vi "_ClassMethodsInheritance_Interface.vi"(9 "EventsIn":T1, 10 "Events":T2) -> ()   [LabVIEW 2013, in "ClassMethodsInheritance.lvclass"]
uses:
  ClassMethodsInheritance.lvclass
  <resource>/Framework/Providers/Veritech_LVCM/Support/Framework/_Plugins/_LVCMPlugin/_LVCMPlugin_EventsOut.ctl
  <resource>/Framework/Providers/Veritech_LVCM/Support/Framework/_Plugins/_LVCMPlugin/_LVCMPlugin_EventsIn.ctl
  <resource>/Framework/Providers/Veritech_LVCM/Support/Framework/_Plugins/_LVCMPlugin/_LVCMPlugin.lvclass
panel:
  in  "Multicolumn Listbox":i32(listbox)
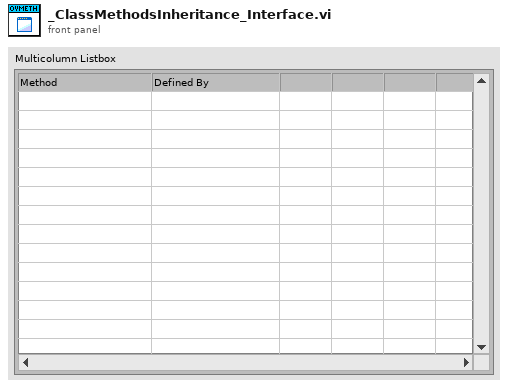
[diagram p1: front panel]
types:
  T1 = typedef "_LVCMPlugin.lvclass/_LVCMPlugin_EventsIn.ctl" = cluster{"Stop":refnum<user-event>, "Activate":refnum<user-event>}
  T2 = typedef "_LVCMPlugin.lvclass/_LVCMPlugin_EventsOut.ctl" = cluster{"ItemEdited":refnum<user-event>}
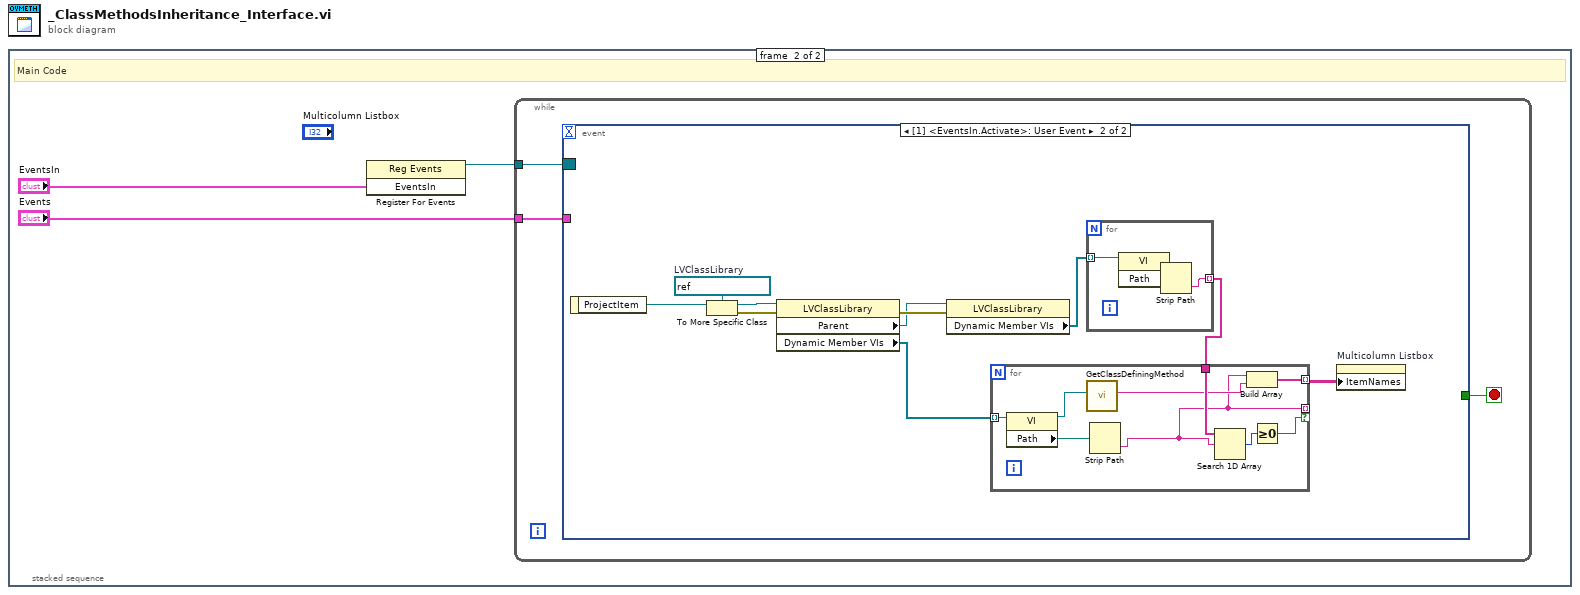
[diagram p0: block diagram]
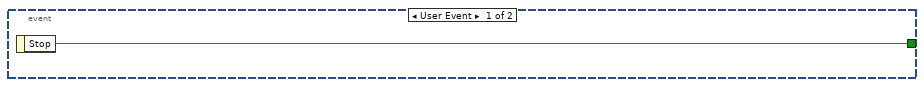
[diagram p3: hidden frame]
diagram:
  n1 = stacked-sequence {
    frame #0 {
      # "Init"
    }
    frame #1 {
      # "Main Code"
      n2 = register-events("EventsIn") -> (reference out=w2:refnum<event-registration>)  [unwired: 2 in, 1 out]
      n3 = while {
        tunnel: w2 -> [w6]
        tunnel: "Events" -> [w5]
        stop <- w4 stop-if-true
        n4 = event shown="[1] <EventsIn.Activate>: User Event" {
          selector: w6 -> [_ _]
          dyn-events: _ -> [_ _]
          timeout: _ -> [_ _]
          tunnel: w5 -> [_ _]
          tunnel: [w7 _] -> w4
          event User Event {
            n5 = event-data() -> ("Stop"=w7:bool)  [unwired: 1 in]
          }
          event User Event {
            w17 = refnum<vi> refnum  # LVClassLibrary
            n6 = event-data() -> ("ProjectItem"=w16:refnum<vi>)  [unwired: 1 in]
            n7 = To More Specific Class(target class=w17, reference=w16) -> (specific class reference=w15:refnum<vi>, error out=w14:errorcluster)  [unwired: 1 in]
            n8 = property class="LVClassLibrary"(reference=w15, error in=w14) -> (error out=w13:errorcluster, "Parent"=w8:refnum<vi>, "Dynamic Member VIs"=w12:refnum<vi>[])  [unwired: 1 out]
            n9 = property class="LVClassLibrary"(reference=w8, error in=w13) -> ("Dynamic Member VIs"=w11:refnum<vi>[])  [unwired: 2 out]
            n10 = for {
              tunnel: w11 -> [w20] mode=indexing
              tunnel: [w18] -> w10 mode=indexing
              n11 = property class="VI"(reference=w20) -> ("Path"=w19:path)  [unwired: 1 in, 2 out]
              n12 = Strip Path(path=w19) -> (name=w18:string)  [unwired: 1 out]
            }
            n13 = for {
              tunnel: w12 -> [w29] mode=indexing
              tunnel: w10 -> [w28]
              tunnel: [w22] -> _ mode=indexing if=w25
              tunnel: [w21] -> w9 mode=indexing
              n14 = property class="VI"(reference=w29) -> (reference out=w24:refnum<vi>, "Path"=w26:path)  [unwired: 1 in, 1 out]
              n15 = call "GetClassDefiningMethod.vi"("MethodVI"=w24) -> ("DefiningClass"=w23:string)  [unwired: 9 in, 1 out]
              n16 = Strip Path(path=w26) -> (name=w22:string)  [unwired: 1 out]
              n17 = Search 1D Array(1D array=w28, element=w22) -> (index of element=w27:i32)  [unwired: 1 in]
              n18 = Build Array(w22, w23) -> (w21:string[])
              n19 = Greater Or Equal To 0?(x=w27) -> (x >= 0?=w25:bool)
            }
            n20 = property on="Multicolumn Listbox" class="MCListbox (strict)"("ItemNames"=w9) -> ()  [unwired: 2 in, 2 out]
          }
        }
      }
    }
  }
